vi "DSF.Engine.Execution.Builder.Set FIFOs.vi"(8 "error in (no error)":errorcluster, 10 "FIFOs":T1, 11 "Builder in":refnum<class "DSF.Engine.Execution.Builder.lvclass">) -> (0 "error out":errorcluster, 3 "Builder out":refnum<class "DSF.Engine.Execution.Builder.lvclass">)   [LabVIEW 2016, in "DSF.Engine.lvlib" / "DSF.Engine.Execution.Builder.lvclass"]
uses:
  DSF.Engine.Execution.Builder.lvclass
  DSF.Engine.Execution.Builder.FIFOs.ctl
  DSF.Engine.Execution.Builder.Command FIFO.ctl
  DSF.Engine.Execution.Builder.Command Payload.ctl
  DSF.Engine.Execution.Builder.Commands.ctl
  DSF.Engine.Execution.Builder.Response FIFO.ctl
  DSF.Engine.Execution.Builder.Response Payload.ctl
  DSF.Engine.Execution.Builder.lvclass/DSF.Engine.Execution.Builder.ctl
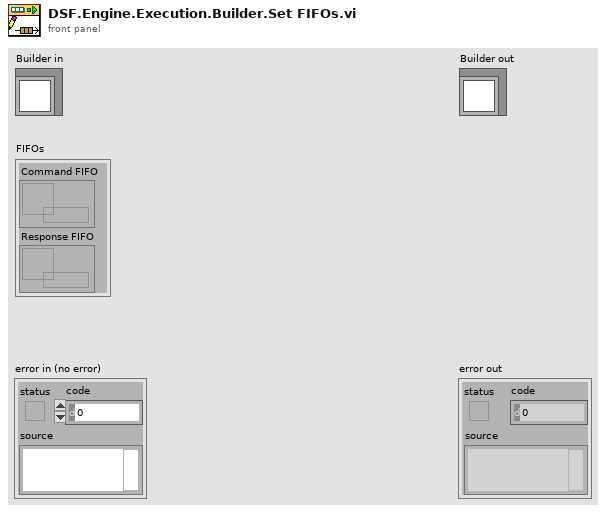
[diagram p1: front panel]
types:
  T1 = typedef "DSF.Engine.lvlib/DSF.Engine.Execution.Builder.lvclass/DSF.Engine.Execution.Builder.FIFOs.ctl" = cluster{"Command FIFO":T2, "Response FIFO":T3}
  T2 = typedef "DSF.Engine.lvlib/DSF.Engine.Execution.Builder.lvclass/DSF.Engine.Execution.Builder.Command FIFO.ctl" = refnum<k33>
  T3 = typedef "DSF.Engine.lvlib/DSF.Engine.Execution.Builder.lvclass/DSF.Engine.Execution.Builder.Response FIFO.ctl" = refnum<k33>
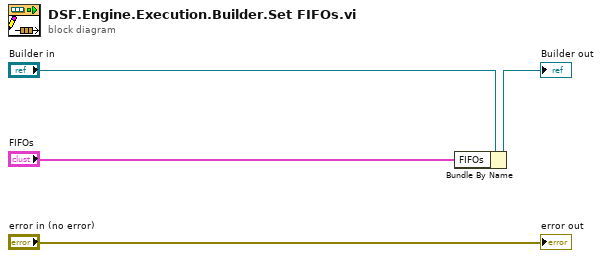
[diagram p0: block diagram]
diagram:
  n1 = Bundle By Name(cluster="Builder in", "FIFOs"="FIFOs") -> (→"Builder out":refnum<class "DSF.Engine.Execution.Builder.lvclass">)
  "error out" <- "error in (no error)"
